vi "CalculatePhase(Host).vi"() -> ()   [LabVIEW 2011]
uses:
  <vilib>/rvi/interface/RandomDataEmulation/nirviRandomDataOpen.vi
  <vilib>/rvi/interface/RandomDataEmulation/nirviRandomDataDMAMethods.vi
  <vilib>/rvi/interface/RandomDataEmulation/niFpgaWriteControlTemplate.vi
  <vilib>/rvi/interface/RandomDataEmulation/niFpgaReadControlTemplate.vi
  <vilib>/rvi/interface/RandomDataEmulation/nirviRandomDataClose.vi
  <vilib>/rvi/interface/nirviOpenFPGA/nirviOpenFPGA.xnode
  <vilib>/rvi/interface/nirviMethod/nirviMethod.xnode
  <vilib>/rvi/interface/nirviReadWriteControl/nirviReadWriteControl.xnode
  <vilib>/rvi/interface/nirviCloseFPGA/nirviCloseFPGA.xnode
panel:
  out "Signal Display":waveform(dbl)[](graph)
  out "Expected Phase Difference":dbl format="%.2f"
  out "Wrrite Overflow":bool
  in  "Phase Offset (periods)":dbl(knob) scale=0.0..1.0
  out "Calculated Phase Difference":dbl
  in  "Stop":bool
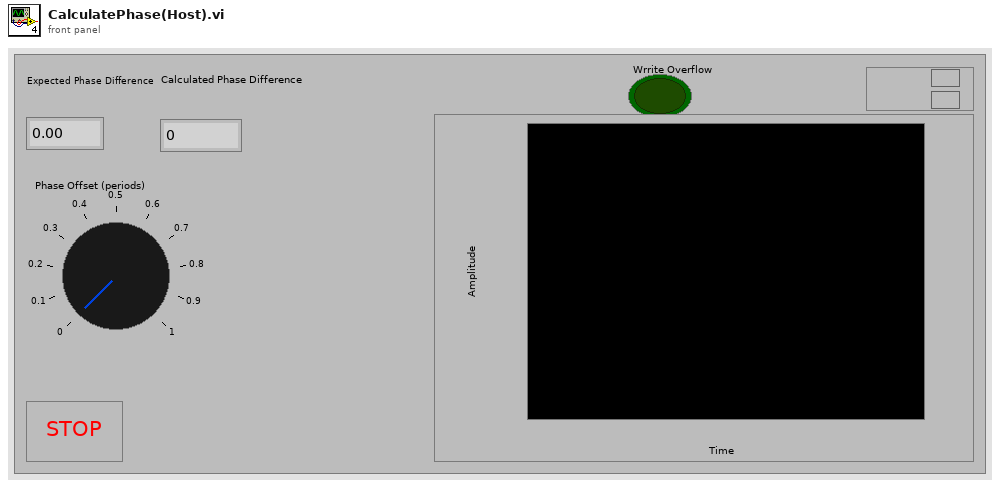
[diagram p1: front panel]
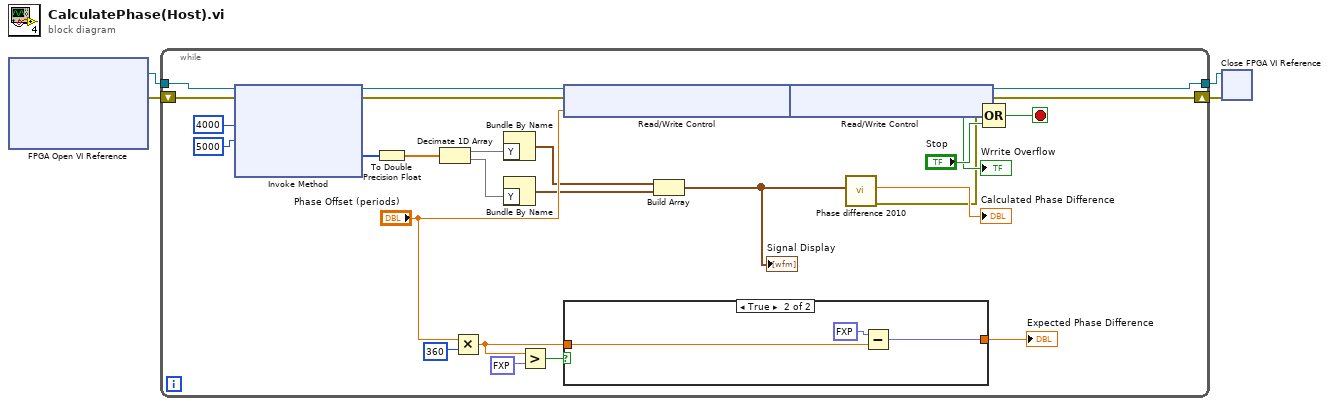
[diagram p0: block diagram]
diagram:
  n1 = xnode "FPGA Open VI Reference"() -> ("FPGA VI Reference Out"=w4:refnum<k20>, "error out"=w3:errorcluster)  [unwired: 2 in]
  n2 = while {
    tunnel: w4 -> [w30]
    shift-right: [w24] -> w2
    shift-left: w3 -> [w28]
    tunnel: [w25] -> w1
    stop <- w32 stop-if-true
    n3 = xnode "Invoke Method"("FPGA VI Reference In"=w30, "error in"=w28, "Number of Elements"=u32 4000, "Timeout (ms)"=5000) -> ("FPGA VI Reference Out"=w12:refnum<k20>, "error out"=w22:errorcluster, "Data"=w19:i16[])  [unwired: 1 out]
    n4 = To Double Precision Float(number=w19) -> (double precision float=w18:dbl[])
    n5 = Decimate 1D Array(w18) -> (w17:dbl[], w16:dbl[])
    n6 = Multiply(x="Phase Offset (periods)", y=360) -> (x*y=w6:dbl)
    n7 = Bundle By Name("Y"=w17) -> (w11:waveform(dbl))  [unwired: 1 in]
    n8 = Bundle By Name("Y"=w16) -> (w10:waveform(dbl))  [unwired: 1 in]
    n9 = Greater?(x=w6, y=fxp<+/-,64,32> 180.0) -> (0:w7:bool)
    n10 = xnode "Read/Write Control"("FPGA VI Reference In"=w12, "error in"=w22, "phase offset (periods)"="Phase Offset (periods)") -> ("FPGA VI Reference Out"=w27:refnum<k20>, "error out"=w26:errorcluster)
    n11 = case shown="True" w7 {
      tunnel: w6 -> [w33 w36]
      tunnel: [w33 w34] -> w5
      frame False {
      }
      frame True {
        n12 = Subtract(x=fxp<+/-,64,32> 360.0, y=w36) -> (x-y=w34:fxp<+/-,64,34>)
      }
    }
    "Expected Phase Difference" <- w5
    n13 = Build Array(w11, w10) -> (w14:waveform(dbl)[])
    "Signal Display" <- w14
    n14 = xnode "Read/Write Control"("FPGA VI Reference In"=w27, "error in"=w26) -> ("FPGA VI Reference Out"=w25:refnum<k20>, "error out"=w24:errorcluster, "Timed Out?"=→"Wrrite Overflow":bool)
    n15 = call "Phase difference 2010.vi"("Signals"=w14) -> ("Max Phase Difference"=→"Calculated Phase Difference":dbl, "Error Out"=w13:errorcluster)  [unwired: 6 in, 2 out]
    n16 = Compound Arithmetic op=OR(w13, w24, "Stop") -> (w32:bool)
  }
  n17 = xnode "Close FPGA VI Reference"("FPGA VI Reference In"=w1, "error in"=w2) -> ()  [unwired: 1 out]
